vi "Update Status Table.vi"(8 "error in (no error)":errorcluster, 10 "error_info":T11[](array[typedef])) -> (0 "error out":errorcluster, 3 "Error MCLB reference out":refnum<vi>)   [LabVIEW 2021, in "CIF_UI.lvclass"]
uses:
  CIF_UI.lvclass
  CIFPluginManager/CIFPluginManager/gRPC/CIF_Manager_client/RPC Messages/cif_manager_ErrorInfo.ctl
  Typedef/Controllers.ctl
  CIFCore/Common/Typedef/gRPC Reported Plugin Status.ctl
  CIFCore/Common/Typedef/Plugin State.ctl
  CIFCore/Common/Typedef/Timing Statistics.ctl
  CIFCore/Common/Typedef/Timing Stats Base.ctl
  CIFCore/Common/Typedef/FIFO Statistics.ctl
  CIFCore/Common/Typedef/Simple Error.ctl
  CIFCore/Common/Typedef/Monitor Doubles.ctl
  CIFCore/Common/Typedef/Monitor U64.ctl
  CIFCore/Common/Typedef/Monitor I64.ctl
  CIFPluginManager/CIFPluginManager/gRPC/CIF_Manager_client/CIF_Manager_client.lvlib
  CIFCore/Common/CIFCoreCommon.lvlib
panel:
  in  "Controller Status":T1[](array[typedef]) {"Status"."Monitor Doubles"."4" format="%#_9g"; "Status"."Monitor Doubles"."3" format="%#_9g"; "Status"."Monitor Doubles"."2" format="%#_9g"; "Status"."Monitor Doubles"."1" format="%#_9g"}
  out "Status Table reference out":refnum<vi>
  in  "Status Table reference in":refnum<vi>
  in  "Table Control":string[][](table)
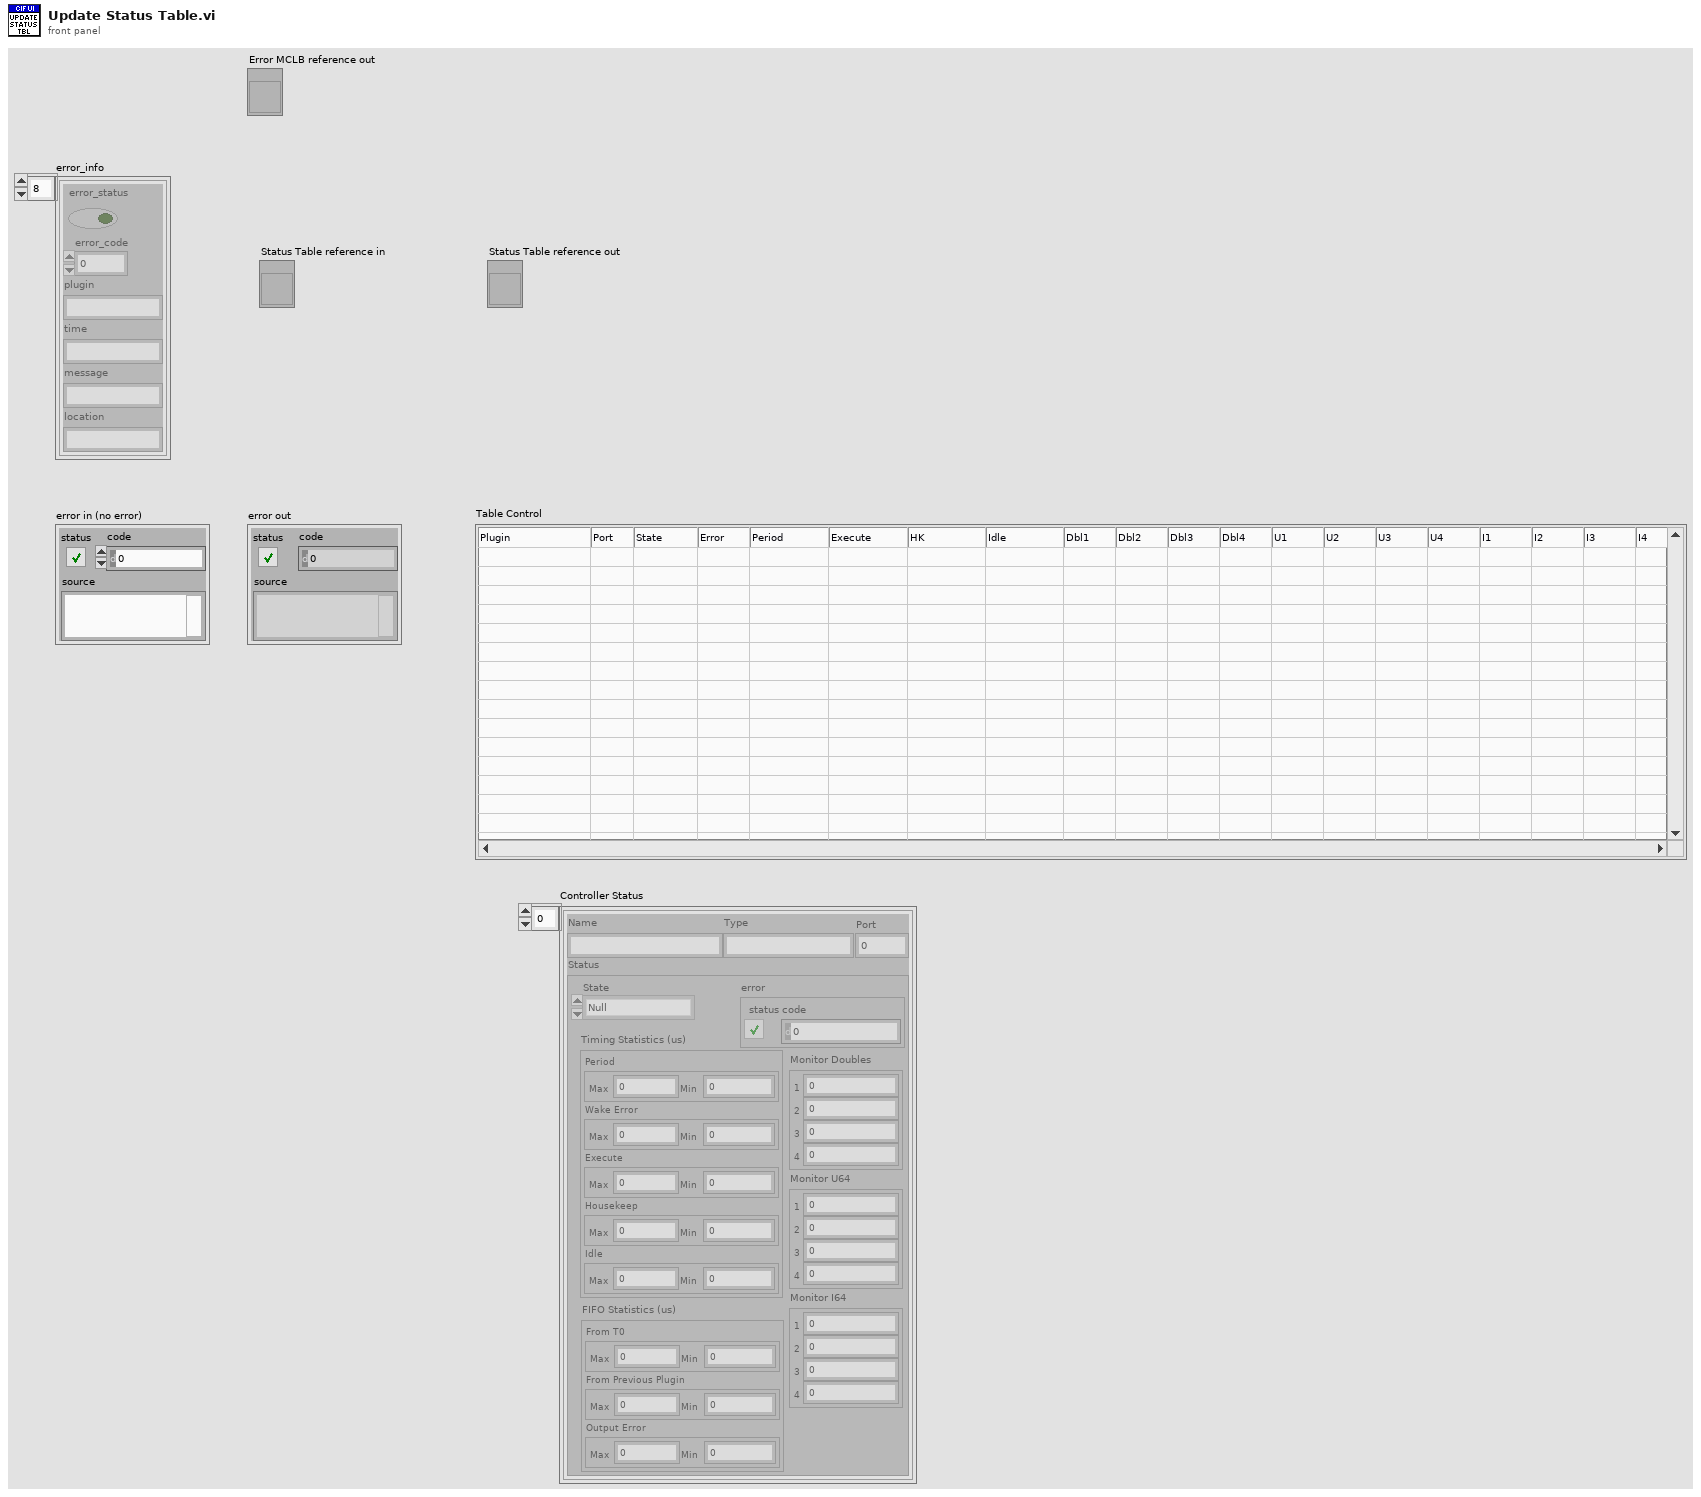
[diagram p1: front panel]
types:
  T1 = typedef "CIF_UI.lvclass/Controllers.ctl" = cluster{"Name":string, "Type":string, "Port":i32, "Status":T2}
  T2 = typedef "CIFCoreCommon.lvlib/gRPC Reported Plugin Status.ctl" = cluster{"State":T3, "Timing Statistics (us)":T4, "FIFO Statistics (us)":T6, "error":T7, "Monitor Doubles":T8, "Monitor U64":T9, "Monitor I64":T10}
  T3 = typedef "CIFCoreCommon.lvlib/Plugin State.ctl" = enum32{"Null", "Creating", "Listening", "Running", "CleaningUp", "Destroying"}
  T4 = typedef "CIFCoreCommon.lvlib/Timing Statistics.ctl" = cluster{"Period":T5, "Wake Error":T5, "Execute":T5, "Housekeep":T5, "Idle":T5}
  T5 = typedef "CIFCoreCommon.lvlib/Timing Stats Base.ctl" = cluster{"Max":i32, "Min":i32}
  T6 = typedef "CIFCoreCommon.lvlib/FIFO Statistics.ctl" = cluster{"From T0":T5, "From Previous Plugin":T5, "Output Error":T5}
  T7 = typedef "CIFCoreCommon.lvlib/Simple Error.ctl" = cluster{"status":bool, "code":i32}
  T8 = typedef "CIFCoreCommon.lvlib/Monitor Doubles.ctl" = cluster{"1":dbl, "2":dbl, "3":dbl, "4":dbl}
  T9 = typedef "CIFCoreCommon.lvlib/Monitor U64.ctl" = cluster{"1":u64, "2":u64, "3":u64, "4":u64}
  T10 = typedef "CIFCoreCommon.lvlib/Monitor I64.ctl" = cluster{"1":i64, "2":i64, "3":i64, "4":i64}
  T11 = typedef "CIF_Manager_client.lvlib/cif_manager_ErrorInfo.ctl" = cluster{"error_status":bool, "error_code":i32, "plugin":string, "time":string, "message":string, "location":string}
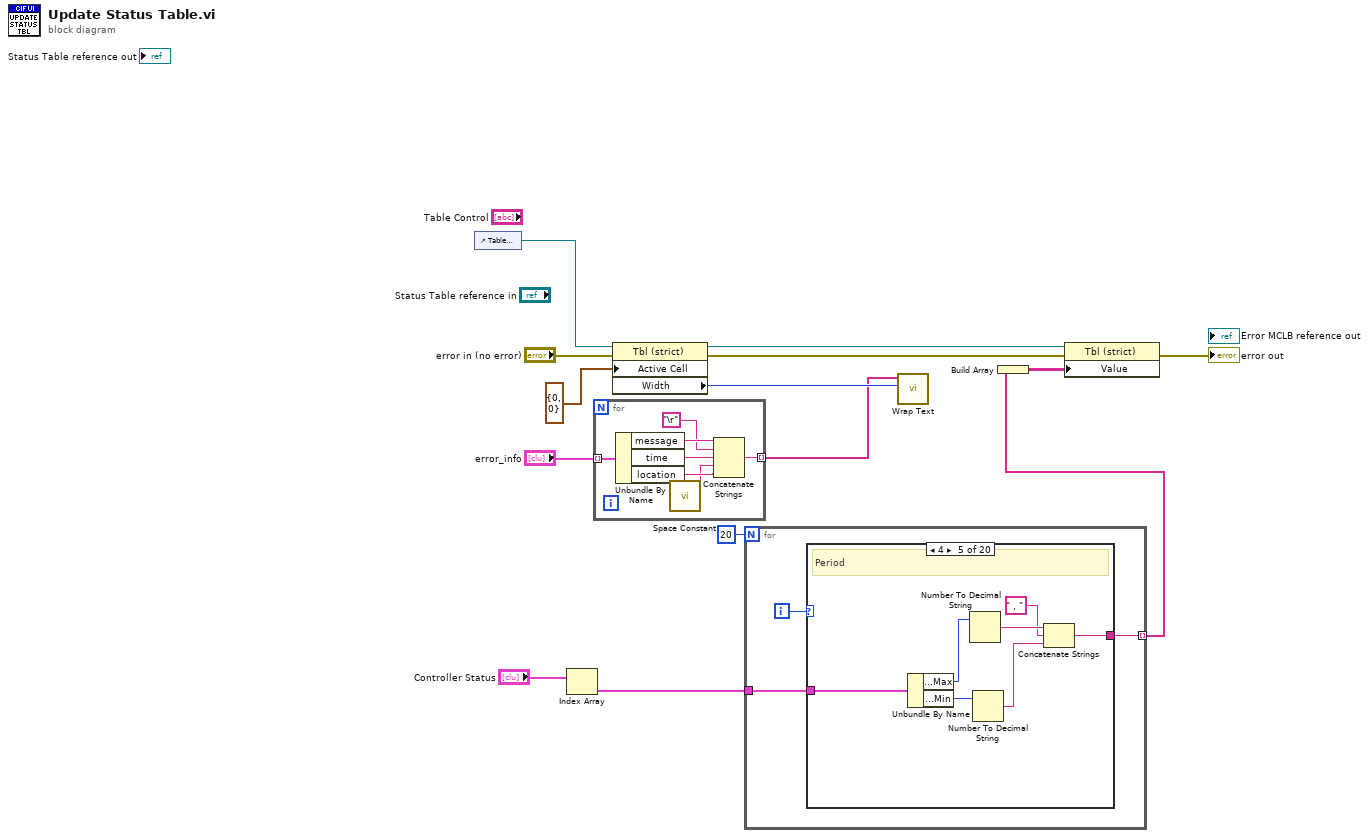
[diagram p0: block diagram]
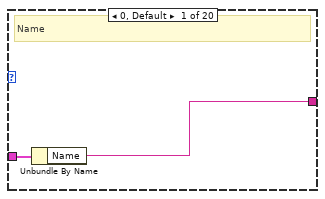
[diagram p2: hidden frame]
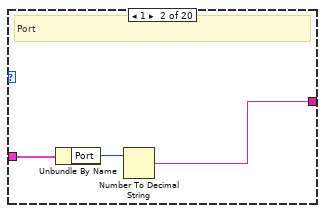
[diagram p3: hidden frame]
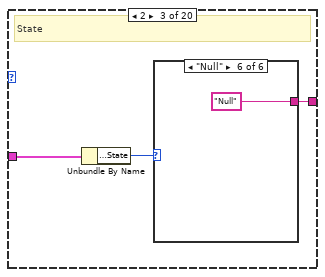
[diagram p4: hidden frame]
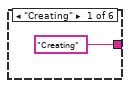
[diagram p5: hidden frame]
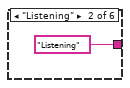
[diagram p6: hidden frame]
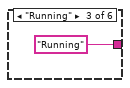
[diagram p7: hidden frame]
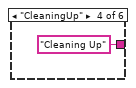
[diagram p8: hidden frame]
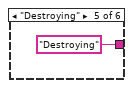
[diagram p9: hidden frame]
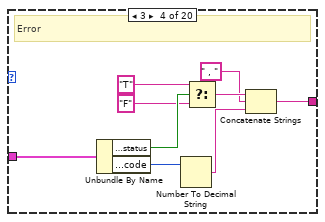
[diagram p10: hidden frame]
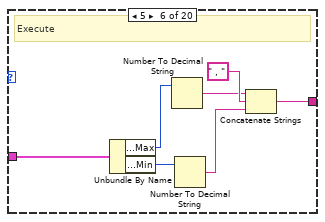
[diagram p11: hidden frame]
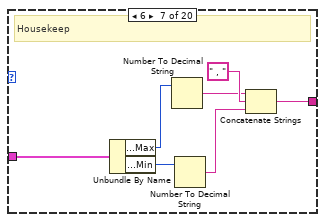
[diagram p12: hidden frame]
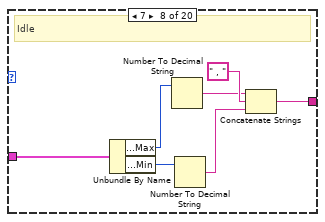
[diagram p13: hidden frame]
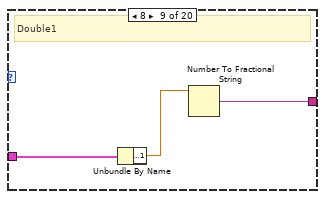
[diagram p14: hidden frame]
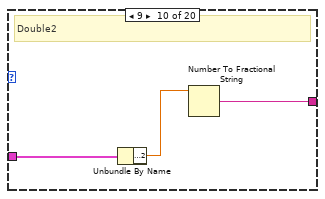
[diagram p15: hidden frame]
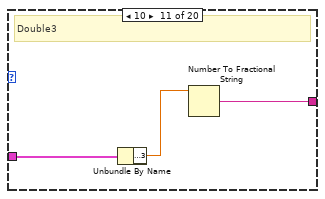
[diagram p16: hidden frame]
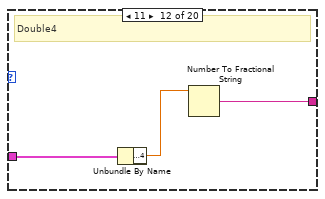
[diagram p17: hidden frame]
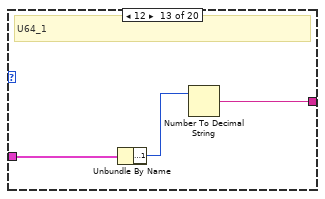
[diagram p18: hidden frame]
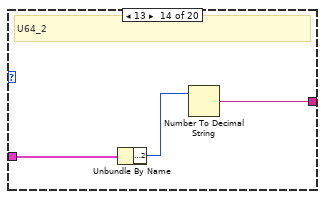
[diagram p19: hidden frame]
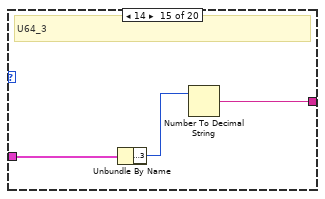
[diagram p20: hidden frame]
diagram:
  n1 = control-ref of="Table Control"() -> (w6:refnum<vi>)
  n2 = Index Array(array="Controller Status") -> (element=w1:T1)  [unwired: 1 in]
  n3 = for {
    tunnel: "error_info" -> [w21] mode=indexing
    tunnel: [w19] -> w11 mode=indexing
    n4 = Unbundle By Name(w21) -> ("message"=w20:string, "time"=w17:string, "location"=w18:string)
    n5 = call <vilib>:"Space Constant.vi"() -> ("String"=w15:string)
    n6 = Concatenate Strings(w20, "\r", w17, w15, w18) -> (w19:string)
  }
  n7 = property on="Property Node" class="Tbl (strict)"(reference=w6, error in="error in (no error)", "Active Cell"=cluster{"Row":i32, "Column":i32} {"Row"=0, "Column"=0}) -> (reference out=w7:refnum<vi>, error out=w8:errorcluster, "Width"=w12:u32)
  n8 = for {
    N: 20 -> [_]
    tunnel: [w23] -> w4 mode=indexing
    tunnel: w1 -> [w22]
    i -> [w24]
    n9 = case shown="4" w24 {
      tunnel: [w25 w29 w30 w39 w51 w57 w64 w71 w76 w79 w82 w85 w88 w91 w94 w97 w100 w103 w106 w109] -> w23
      tunnel: w22 -> [w26 w28 w32 w47 w54 w61 w68 w75 w78 w81 w84 w87 w90 w93 w96 w99 w102 w105 w108 w111]
      frame 0, Default {
        # "Name"
        n10 = Unbundle By Name(w26) -> ("Name"=w25:string)
      }
      frame 1 {
        # "Port"
        n11 = Unbundle By Name(w28) -> ("Port"=w27:i32)
        n12 = Number To Decimal String(number=w27) -> (decimal integer string=w29:string)  [unwired: 1 in]
      }
      frame 2 {
        # "State"
        n13 = Unbundle By Name(w32) -> ("Status.State"=w31:T3)
        n14 = case shown="\"Null\"" w31 {
          tunnel: ["Creating" "Listening" "Running" "Cleaning Up" "Destroying" "Null"] -> w30
          frame "Creating" {
          }
          frame "Listening" {
          }
          frame "Running" {
          }
          frame "CleaningUp" {
          }
          frame "Destroying" {
          }
          frame "Null" {
          }
        }
      }
      frame 3 {
        # "Error"
        n15 = Unbundle By Name(w47) -> ("Status.error.status"=w45:bool, "Status.error.code"=w46:i32)
        n16 = Number To Decimal String(number=w46) -> (decimal integer string=w40:string)  [unwired: 1 in]
        n17 = Select(t="T", s=w45, f="F") -> (s? t:f=w42:string)
        n18 = Concatenate Strings(w42, " , ", w40) -> (w39:string)
      }
      frame 4 {
        # "Period"
        n19 = Unbundle By Name(w54) -> ("Status.Timing Statistics (us).Period.Max"=w50:i32, "Status.Timing Statistics (us).Period.Min"=w53:i32)
        n20 = Number To Decimal String(number=w50) -> (decimal integer string=w49:string)  [unwired: 1 in]
        n21 = Number To Decimal String(number=w53) -> (decimal integer string=w52:string)  [unwired: 1 in]
        n22 = Concatenate Strings(w49, " , ", w52) -> (w51:string)
      }
      frame 5 {
        # "Execute"
        n23 = Unbundle By Name(w61) -> ("Status.Timing Statistics (us).Execute.Max"=w56:i32, "Status.Timing Statistics (us).Execute.Min"=w60:i32)
        n24 = Number To Decimal String(number=w56) -> (decimal integer string=w55:string)  [unwired: 1 in]
        n25 = Number To Decimal String(number=w60) -> (decimal integer string=w58:string)  [unwired: 1 in]
        n26 = Concatenate Strings(w55, " , ", w58) -> (w57:string)
      }
      frame 6 {
        # "Housekeep"
        n27 = Unbundle By Name(w68) -> ("Status.Timing Statistics (us).Housekeep.Max"=w63:i32, "Status.Timing Statistics (us).Housekeep.Min"=w67:i32)
        n28 = Number To Decimal String(number=w63) -> (decimal integer string=w62:string)  [unwired: 1 in]
        n29 = Number To Decimal String(number=w67) -> (decimal integer string=w65:string)  [unwired: 1 in]
        n30 = Concatenate Strings(w62, " , ", w65) -> (w64:string)
      }
      frame 7 {
        # "Idle"
        n31 = Unbundle By Name(w75) -> ("Status.Timing Statistics (us).Idle.Max"=w70:i32, "Status.Timing Statistics (us).Idle.Min"=w74:i32)
        n32 = Number To Decimal String(number=w70) -> (decimal integer string=w69:string)  [unwired: 1 in]
        n33 = Number To Decimal String(number=w74) -> (decimal integer string=w72:string)  [unwired: 1 in]
        n34 = Concatenate Strings(w69, " , ", w72) -> (w71:string)
      }
      frame 8 {
        # "Double1"
        n35 = Unbundle By Name(w78) -> ("Status.Monitor Doubles.1"=w77:dbl)
        n36 = Number To Fractional String(number=w77) -> (F-format string=w76:string)  [unwired: 3 in]
      }
      frame 9 {
        # "Double2"
        n37 = Unbundle By Name(w81) -> ("Status.Monitor Doubles.2"=w80:dbl)
        n38 = Number To Fractional String(number=w80) -> (F-format string=w79:string)  [unwired: 3 in]
      }
      frame 10 {
        # "Double3"
        n39 = Unbundle By Name(w84) -> ("Status.Monitor Doubles.3"=w83:dbl)
        n40 = Number To Fractional String(number=w83) -> (F-format string=w82:string)  [unwired: 3 in]
      }
      frame 11 {
        # "Double4"
        n41 = Unbundle By Name(w87) -> ("Status.Monitor Doubles.4"=w86:dbl)
        n42 = Number To Fractional String(number=w86) -> (F-format string=w85:string)  [unwired: 3 in]
      }
      frame 12 {
        # "U64_1"
        n43 = Unbundle By Name(w90) -> ("Status.Monitor U64.1"=w89:u64)
        n44 = Number To Decimal String(number=w89) -> (decimal integer string=w88:string)  [unwired: 1 in]
      }
      frame 13 {
        # "U64_2"
        n45 = Unbundle By Name(w93) -> ("Status.Monitor U64.2"=w92:u64)
        n46 = Number To Decimal String(number=w92) -> (decimal integer string=w91:string)  [unwired: 1 in]
      }
      frame 14 {
        # "U64_3"
        n47 = Unbundle By Name(w96) -> ("Status.Monitor U64.3"=w95:u64)
        n48 = Number To Decimal String(number=w95) -> (decimal integer string=w94:string)  [unwired: 1 in]
      }
      frame 15 {
        # "U64_4"
        n49 = Unbundle By Name(w99) -> ("Status.Monitor U64.4"=w98:u64)
        n50 = Number To Decimal String(number=w98) -> (decimal integer string=w97:string)  [unwired: 1 in]
      }
      frame 16 {
        # "I64_1"
        n51 = Unbundle By Name(w102) -> ("Status.Monitor I64.1"=w101:i64)
        n52 = Number To Decimal String(number=w101) -> (decimal integer string=w100:string)  [unwired: 1 in]
      }
      frame 17 {
        # "I64_2"
        n53 = Unbundle By Name(w105) -> ("Status.Monitor I64.2"=w104:i64)
        n54 = Number To Decimal String(number=w104) -> (decimal integer string=w103:string)  [unwired: 1 in]
      }
      frame 18 {
        # "I64_3"
        n55 = Unbundle By Name(w108) -> ("Status.Monitor I64.3"=w107:i64)
        n56 = Number To Decimal String(number=w107) -> (decimal integer string=w106:string)  [unwired: 1 in]
      }
      frame 19 {
        # "I64_4"
        n57 = Unbundle By Name(w111) -> ("Status.Monitor I64.4"=w110:i64)
        n58 = Number To Decimal String(number=w110) -> (decimal integer string=w109:string)  [unwired: 1 in]
      }
    }
  }
  n59 = call "Wrap Text.vi"("width"=w12, "item names"=w11) -> ()  [unwired: 8 in, 2 out]
  n60 = Build Array(w4) -> (w3:string[][])
  n61 = property class="Tbl (strict)"(reference=w7, error in=w8, "Value"=w3) -> (error out=→"error out":errorcluster)  [unwired: 1 out]
